vi "Instrument Manager Loop.vi"(8 "System Control":refnum<queue>, 11 "Instrument Manager":refnum<queue>) -> (0 "error out":errorcluster)   [LabVIEW 2020, in "plugin_flodx_ph_probe.lvlib" / "plugin.lvlib" / "Instrument Manager.lvlib"]
uses:
  Instrument Manager.lvlib
  <userlib>/RxnRover/PluginCore/src/support/Message Queue/Message Cluster.ctl
  Instrument Loop State.ctl
  connection_info/Connection Info.ctl
  Instrument State.ctl
  Instrument Config.ctl
  <vilib>/Utility/error.llb/Error Cluster From Error Code.vi
  <vilib>/ErrorRing/Error Ring.xnode
  <userlib>/RxnRover/PluginCore/src/support/Message Queue/Message Queue.lvlib
  <userlib>/_OpenG.lib/lvdata/lvdata.llb/openg_variant.lvlib
  mock_driver/mock_driver.lvlib
  <instrlib>/RxnRover/FloDx Ph Probe Driver/driver_flodx_ph_probe.lvlib
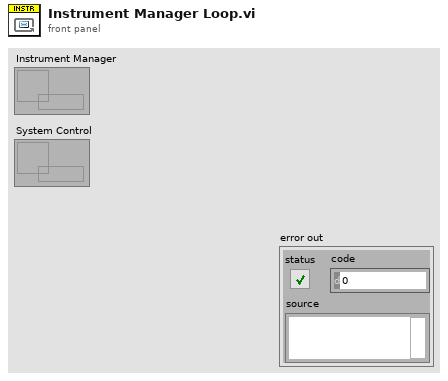
[diagram p1: front panel]
types:
  T1 = typedef "plugin_flodx_ph_probe.lvlib/plugin.lvlib/Instrument Manager.lvlib/Instrument Loop State.ctl" = cluster{"Connection Info":T2, "Running":bool, "Running Since":timestamp, "Instrument State":T3}
  T2 = typedef "plugin_flodx_ph_probe.lvlib/plugin.lvlib/Instrument Manager.lvlib/Connection Info.ctl" = cluster{"VISA Resource":refnum<visa-resource-name>, "Address":u8}
  T3 = typedef "plugin_flodx_ph_probe.lvlib/plugin.lvlib/Instrument Manager.lvlib/Instrument State.ctl" = cluster{"pH":sgl, "Temperature (C)":sgl, "Device":string, "Firmware Version":string, "Error Status":bool, "Error Code":i32, "Error Source":string}
  T4 = typedef "plugin_flodx_ph_probe.lvlib/plugin.lvlib/Instrument Manager.lvlib/Instrument Config.ctl" = cluster{"Address":dbl, "Device":string, "Firmware Version":string}
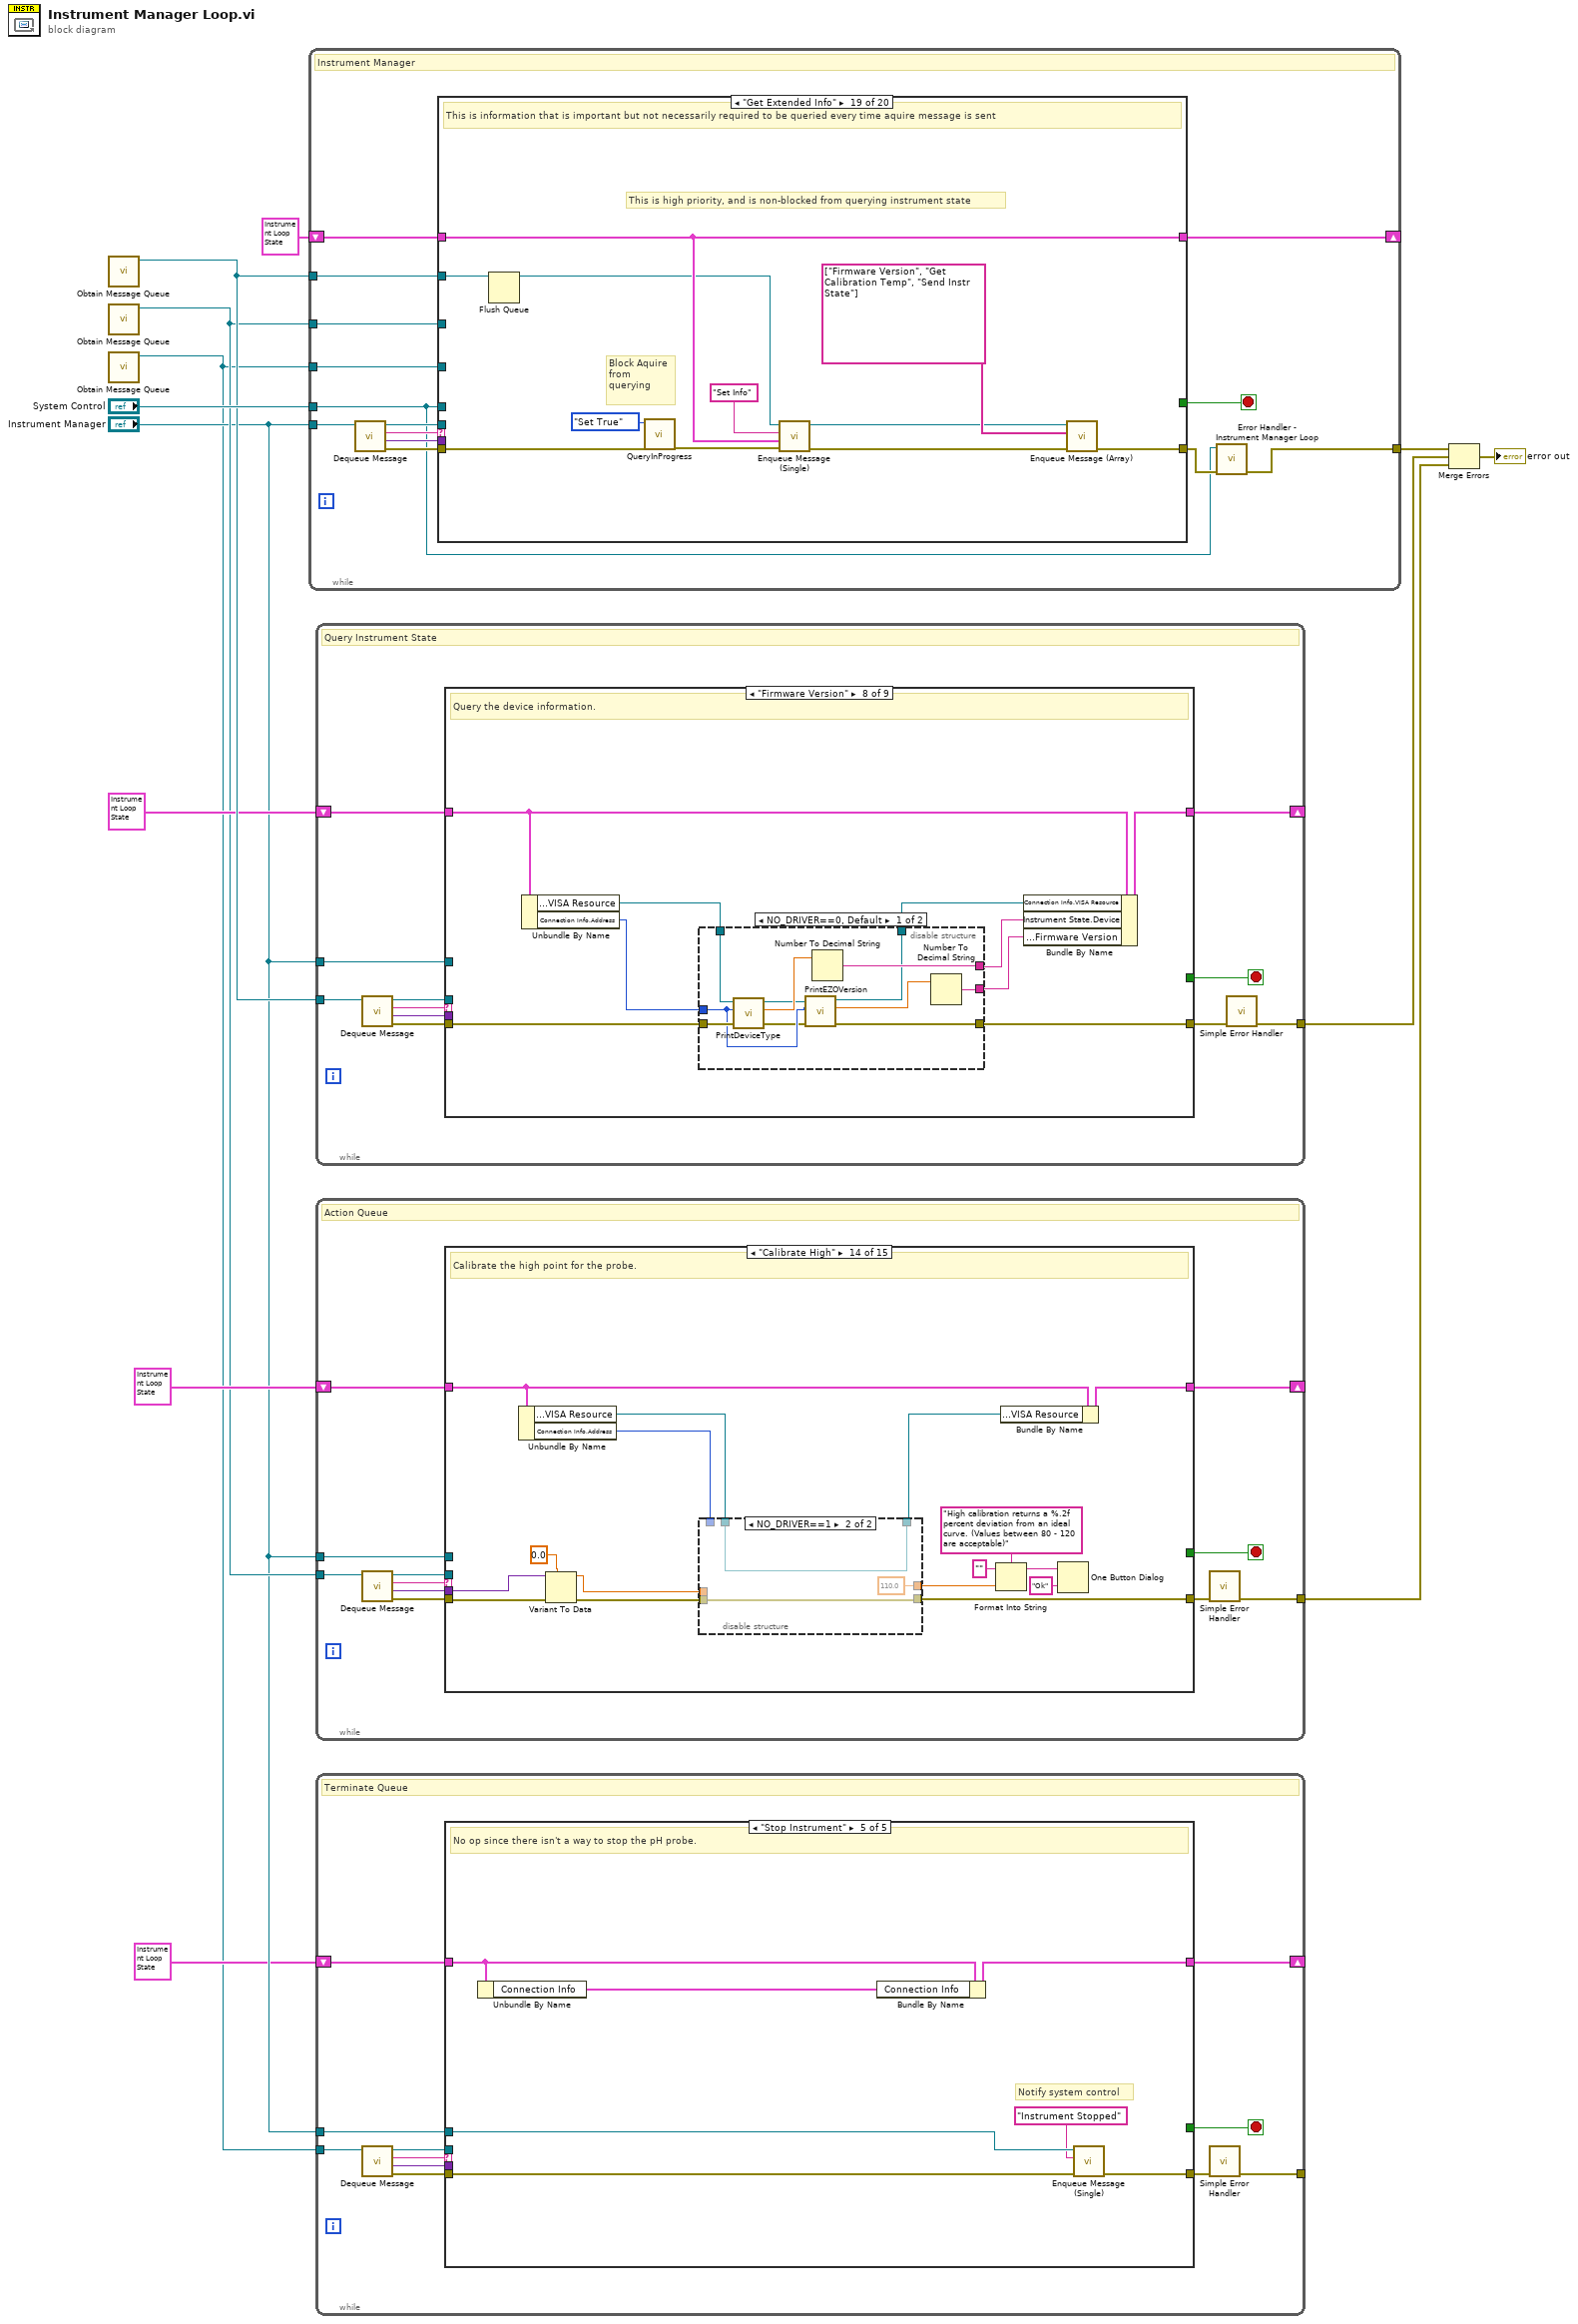
[diagram p0: block diagram]
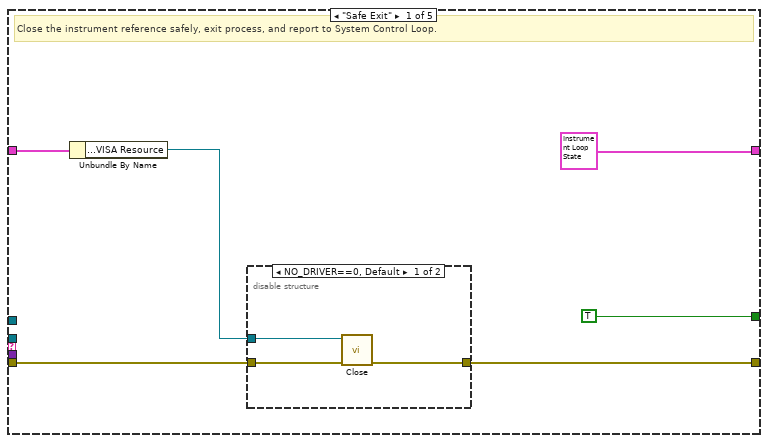
[diagram p2: hidden frame]
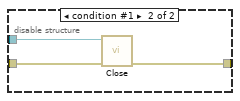
[diagram p3: hidden frame]
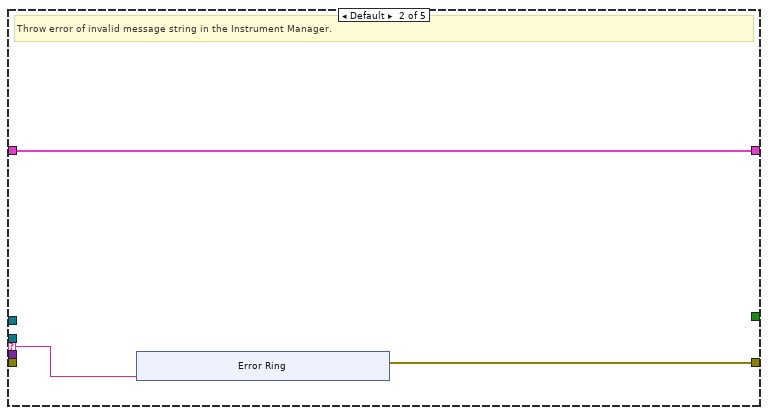
[diagram p4: hidden frame]
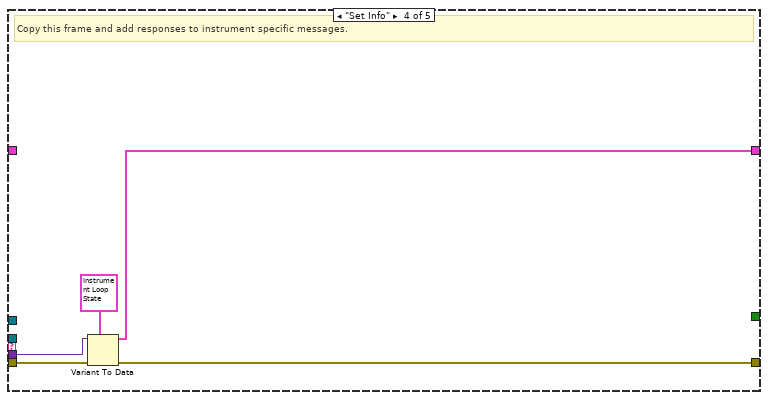
[diagram p6: hidden frame]
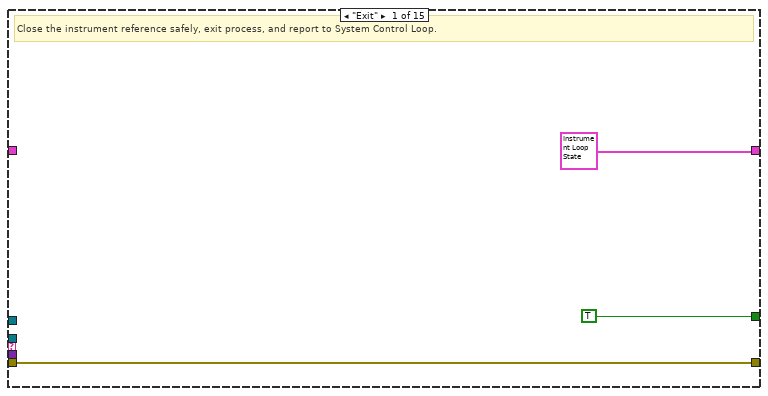
[diagram p7: hidden frame]
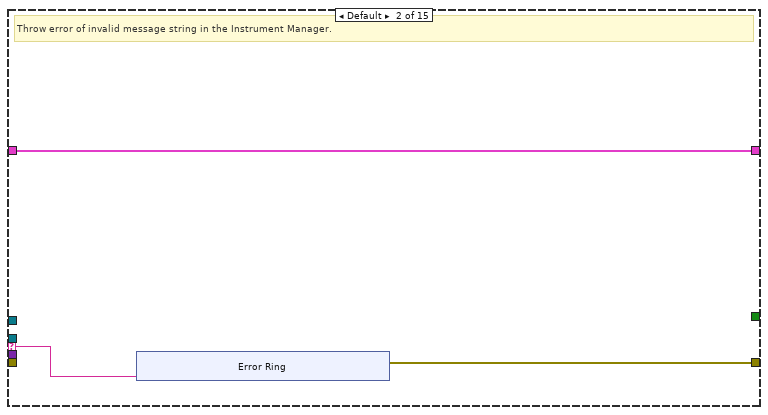
[diagram p8: hidden frame]
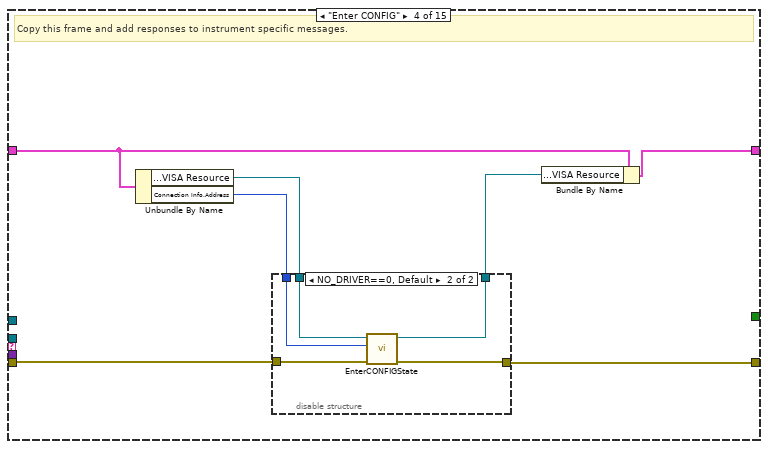
[diagram p10: hidden frame]
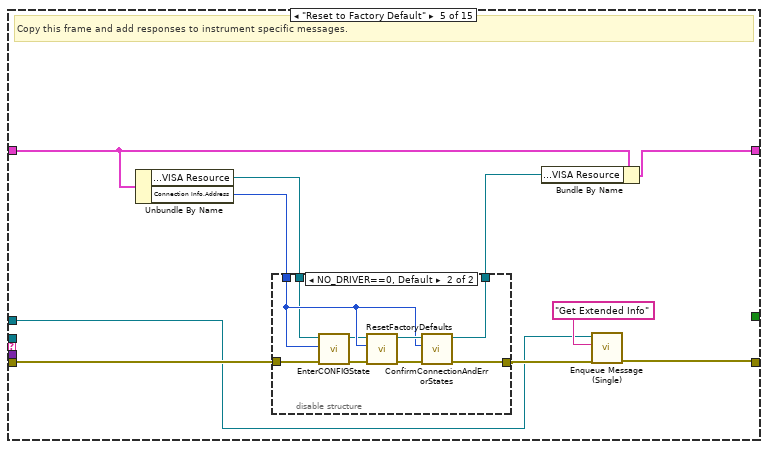
[diagram p12: hidden frame]
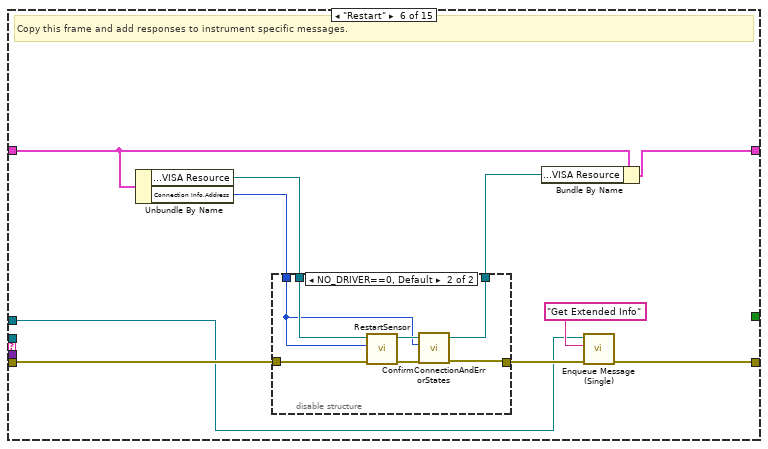
[diagram p14: hidden frame]
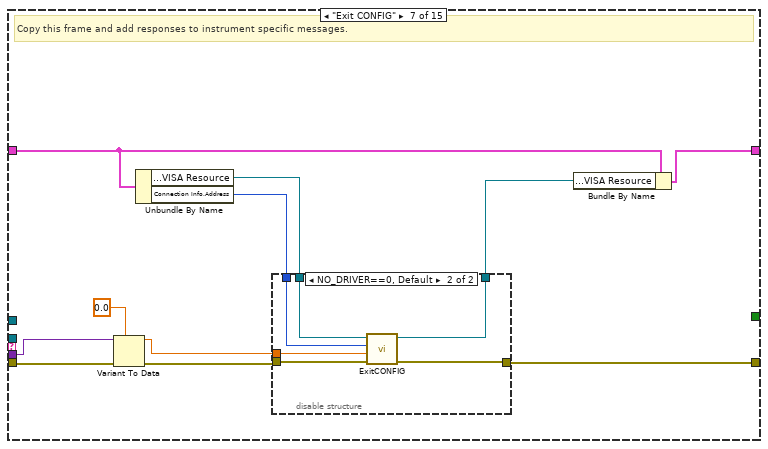
[diagram p16: hidden frame]
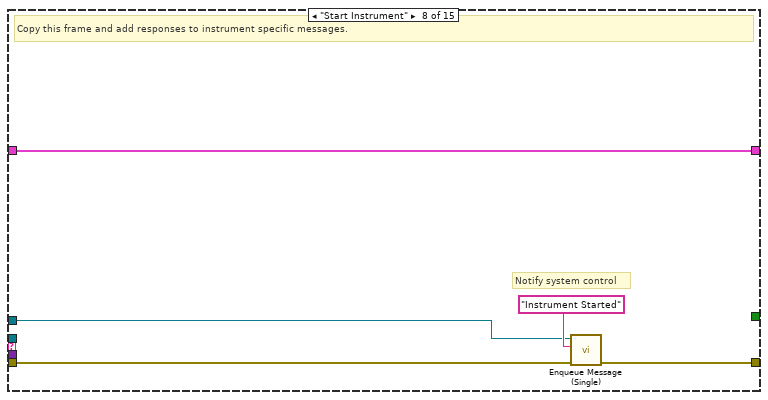
[diagram p18: hidden frame]
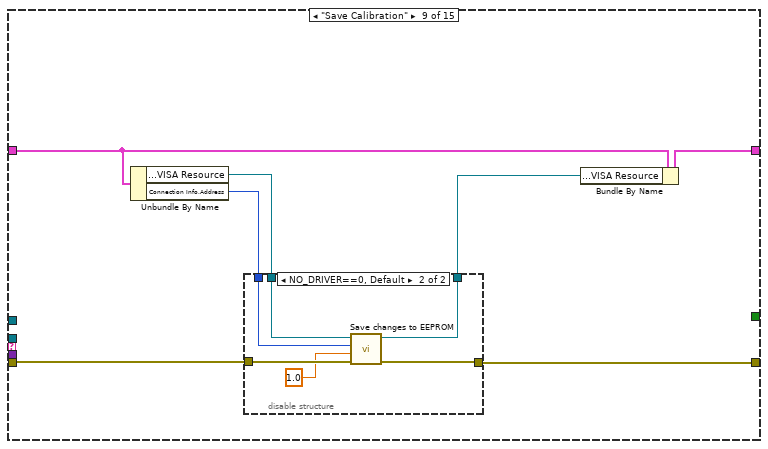
[diagram p19: hidden frame]
diagram:
  n1 = call <userlib>:"Obtain Message Queue.vi"() -> ("Message Queue"=w10:refnum<queue>)  [unwired: 10 in, 1 out]
  n2 = call <userlib>:"Obtain Message Queue.vi"() -> ("Message Queue"=w5:refnum<queue>)  [unwired: 10 in, 1 out]
  n3 = call <userlib>:"Obtain Message Queue.vi"() -> ("Message Queue"=w1:refnum<queue>)  [unwired: 10 in, 1 out]
  n4 = while {
    tunnel: "Instrument Manager" -> [w27]
    tunnel: "System Control" -> [w18]
    tunnel: [w21] -> w13
    shift-right: [w14] -> _
    shift-left: T1 {"Connection Info"={"VISA Resource"="", "Address"=0}, "Running"=FALSE, "Running Since"=timestamp(0 s since 1904-01-01), "Instrument State"={"pH"=0.0, "Temperature (C)"=0.0, "Device"="", "Firmware Version"="", "Error Status"=FALSE, "Error Code"=0, "Error Source"=""}} ("Default Instrument State") -> [w20]
    tunnel: w10 -> [w17]
    tunnel: w5 -> [w16]
    tunnel: w1 -> [w15]
    stop <- w19 stop-if-true
    # "Instrument Manager"
    n5 = call <userlib>:"Dequeue Message.vi"("Message Queue"=w27) -> ("error out"=w23:errorcluster, "Message Data"=w24:variant, "Message"=w26:string, "dup Message Queue"=w25:refnum<queue>)  [unwired: 7 in]
    n6 = case shown="\"Get Extended Info\"" w26 {
      selector: w26 -> [_ w37 _ _ _ _ _ w83 _ _ w128 w132 w145 w154 w164 w176 _ _ _ _]
      tunnel: w25 -> [w30 _ _ w54 _ _ _ _ _ w94 _ _ _ _ _ w174 _ _ _ w215]
      tunnel: w18 -> [_ w38 _ _ w64 w74 w80 _ _ w96 w124 _ _ _ _ _ _ _ _ _]
      tunnel: w24 -> [_ _ _ w61 _ _ _ _ _ w102 w127 w139 w151 w160 w170 w182 _ _ _ w216]
      tunnel: w23 -> [w31 w39 w46 w59 w66 w71 w77 _ w92 w101 w126 w136 w148 w157 w167 w179 w184 w185 w201 w221]
      tunnel: [w29 w33 w47 w56 w65 w75 w81 w82 w92 w105 w129 w140 w152 w161 w162 w172 w184 w191 w211 w212] -> w22
      tunnel: w20 -> [_ w36 _ w60 w67 w69 w78 w84 w93 w104 w125 w137 w149 w158 w168 w180 w183 w190 w208 w220]
      tunnel: [w32 w36 T1 {"Connection Info"={"VISA Resource"="", "Address"=0}, "Running"=FALSE, "Running Since"=timestamp(0 s since 1904-01-01), "Instrument State"={"pH"=0.0, "Temperature (C)"=0.0, "Device"="", "Firmware Version"="", "Error Status"=FALSE, "Error Code"=0, "Error Source"=""}} w60 w67 w69 w78 w84 w93 w103 w125 w131 w144 w158 w168 w180 w183 w190 w208 w214] -> w14
      tunnel: [_ _ TRUE _ _ _ _ _ _ _ _ _ _ _ _ _ _ _ _ _] -> w19
      tunnel: w17 -> [_ _ w41 _ _ _ _ _ _ _ _ _ _ _ _ _ _ w189 w203 _]
      tunnel: w16 -> [_ _ w42 _ _ _ _ _ _ _ _ _ w141 w153 w163 w175 _ _ _ _]
      tunnel: w15 -> [_ _ w43 _ _ _ _ _ _ _ _ w134 _ _ _ _ _ _ _ _]
      frame "Initialize" {
        (unwired) string[] ["Send Instrument Config", "Send Entry Names"]
        w32 = T1 {"Connection Info"={"VISA Resource"="", "Address"=0}, "Running"=FALSE, "Running Since"=timestamp(0 s since 1904-01-01), "Instrument State"={"pH"=0.0, "Temperature (C)"=0.0, "Device"="", "Firmware Version"="", "Error Status"=FALSE, "Error Code"=0, "Error Source"=""}}  # Default Instrument State
        # "Initialize the loop data."
        n7 = call <userlib>:"Enqueue Message (Array).vi"("error in (no error)"=w31, "Message Array"=string[] ["Send Instrument Config", "Send Acquisition Messages", "Send Entry Names"], "Message Queue"=w30) -> ("error out"=w29:errorcluster)  [unwired: 7 in, 1 out]
      }
      frame "Report" {
        # "Unblock querying"
        # "Report the instrument state."
        n8 = call <userlib>:"Enqueue Message (Single).vi"("error in (no error)"=w39, "Message Data"=w36, "Message"=w37, "Message Queue"=w38) -> ("error out"=w34:errorcluster)  [unwired: 6 in, 1 out]
        n9 = call "QueryInProgress.vi"("error in (no error)"=w34, "Action"=enum16{"Get", "Set False", "Set True"}."Set False") -> ("error out"=w33:errorcluster)  [unwired: 8 in, 1 out]
      }
      frame "Exit" {
        # "Close the instrument reference safely, exit process, and report to System Control Loop."
        n10 = Build Array(w41, w42) -> (w40:refnum<queue>[])
        n11 = call <userlib>:"Enqueue Message (Single).vi"("error in (no error)"=w46, "Message"="Safe Exit", "Message Queue"=w43) -> ("error out"=w45:errorcluster)  [unwired: 7 in, 1 out]
        n12 = for {
          tunnel: w40 -> [w52] mode=indexing
          tunnel: w45 -> [w50]
          tunnel: [w53] -> w47
          n13 = call <userlib>:"Enqueue Message (Single).vi"("error in (no error)"=w50, "Message"="Exit", "Message Queue"=w52) -> ("error out"=w53:errorcluster)  [unwired: 7 in, 1 out]
        }
      }
      frame "New Instrument Config" {
        # "No settings right now"
        # "#todo: What if values are invalid? Create \"Invalid Instrument Config\" message maybe."
        # "If the new config is accepted, notify everything of the new values"
        # "Update the configs based on the user settings."
        n14 = Variant To Data(error in=w59, type=T4 {"Address"=0.0, "Device"="", "Firmware Version"=""} ("Instrument Configuration"), Variant=w61) -> (error out=w55:errorcluster)  [unwired: 1 out]
        n15 = call <userlib>:"Enqueue Message (Single).vi"("error in (no error)"=w55, "Message"="Send Instrument Config", "Message Queue"=w54) -> ("error out"=w56:errorcluster)  [unwired: 7 in, 1 out]
      }
      frame "Send Instrument Config" {
        # "Send out the current values for the public loop configs."
        n16 = call <userlib>:"Enqueue Message (Single).vi"("error in (no error)"=w66, "Message Data"=T4 {"Address"=0.0, "Device"="", "Firmware Version"=""} ("Instrument Configuration"), "Message"="Instrument Config", "Message Queue"=w64) -> ("error out"=w65:errorcluster)  [unwired: 6 in, 1 out]
      }
      frame "Send Entry Names" {
        # "#note: This is auto-populated based on the Instrument State TypeDef entry labels."
        # "Send the display names of entry values that will be reported by this instrument in each \"Report\" call."
        n17 = Unbundle By Name(w69) -> ("Instrument State"=w68:T3)
        n18 = call <userlib>:"Get Cluster Element Names__ogtk.vi"("error in (no error)"=w71, "Cluster"=w68) -> ("error out"=w70:errorcluster, "Element Names"=w72:string[])  [unwired: 8 in]
        n19 = call <userlib>:"Enqueue Message (Single).vi"("error in (no error)"=w70, "Message Data"=w72, "Message"="Set Entry Names", "Message Queue"=w74) -> ("error out"=w75:errorcluster)  [unwired: 6 in, 1 out]
      }
      frame "Send Acquisition Messages" {
        # "Send the messages that should be used to acquire the relevant instrument state and how to report it."
        n20 = call <userlib>:"Enqueue Message (Single).vi"("error in (no error)"=w77, "Message Data"=string[] ["Acquire"], "Message"="Set Acquisition Messages", "Message Queue"=w80) -> ("error out"=w81:errorcluster)  [unwired: 6 in, 1 out]
      }
      frame Default {
        # "Throw error of invalid message string in the Instrument Manager."
        n21 = xnode "Error Ring"("parameter 0"=w83) -> ("error out"=w82:errorcluster)
      }
      frame "--- Copy This Frame ---" {
        # "Copy this frame and add responses to instrument specific messages."
      }
      frame "Set Connection Info" {
        # "Validate and initialize the connection info"
        n22 = Variant To Data(error in=w101, type=T2 {"VISA Resource"="", "Address"=0} ("Connection Info"), Variant=w102) -> (data=w99:T2, error out=w100:errorcluster)
        n23 = call "Attempt Connection.vi"("error in (no error)"=w100, "Connection Info"=w99) -> ("error out"=w97:errorcluster, "Connection Info (duplicate)"=w98:T2)  [unwired: 8 in]
        n24 = case shown="No Error" w97 {
          selector: w97 -> [w107 w119]
          tunnel: w98 -> [w106 _]
          tunnel: [w108 w122] -> w105
          tunnel: w104 -> [w115 w123]
          tunnel: [w117 w123] -> w103
          tunnel: w96 -> [w116 w121]
          tunnel: w94 -> [w112 _]
          frame No Error {
            # "Notify System Control of valid connection info"
            # "Initialize valid resource."
            n25 = call <userlib>:"Enqueue Message (Single).vi"("error in (no error)"=w107, "Message Data"=w106, "Message"="Valid Connection Info", "Message Queue"=w116) -> ("error out"=w114:errorcluster)  [unwired: 6 in, 1 out]
            n26 = Bundle By Name(cluster=w115, "Connection Info"=w106) -> (w117:T1)
            n27 = call <userlib>:"Enqueue Message (Single).vi"("error in (no error)"=w114, "Message"="Send Acquisition Messages", "Message Queue"=w112) -> ("error out"=w109:errorcluster, "dup Message Queue"=w111:refnum<queue>)  [unwired: 7 in]
            n28 = call <userlib>:"Enqueue Message (Single).vi"("error in (no error)"=w109, "Message"="Get Extended Info", "Message Queue"=w111) -> ("error out"=w108:errorcluster)  [unwired: 7 in, 1 out]
          }
          frame Error {
            # "Report invalid resource."
            n29 = call <userlib>:"Enqueue Message (Single).vi"("Message Data"=w119, "Message"="Invalid Connection Info", "Message Queue"=w121) -> ("error out"=w122:errorcluster)  [unwired: 7 in, 1 out]
          }
        }
      }
      frame "Instrument Started", "Instrument Stopped" {
        # "Forward start/stop messages to the rest of the program."
        n30 = call <userlib>:"Enqueue Message (Single).vi"("error in (no error)"=w126, "Message Data"=w127, "Message"=w128, "Message Queue"=w124) -> ("error out"=w129:errorcluster)  [unwired: 6 in, 1 out]
      }
      frame "Stop Instrument" {
        # "Stop the instrument action."
        n31 = call <userlib>:"Enqueue Message (Single).vi"("error in (no error)"=w136, "Message Data"=w137, "Message"="Set Info", "Message Queue"=w134) -> ("error out"=w135:errorcluster, "dup Message Queue"=w133:refnum<queue>)  [unwired: 6 in]
        n32 = call <userlib>:"Enqueue Message (Single).vi"("error in (no error)"=w135, "Message Data"=w139, "Message"=w132, "Message Queue"=w133) -> ("error out"=w140:errorcluster)  [unwired: 6 in, 1 out]
        n33 = Bundle By Name(cluster=w137, "Running"=FALSE) -> (w131:T1)
      }
      frame "Start Instrument" {
        # "Start the instrument action."
        n34 = call <userlib>:"Enqueue Message (Single).vi"("error in (no error)"=w148, "Message Data"=w149, "Message"="Set Info", "Message Queue"=w141) -> ("error out"=w147:errorcluster, "dup Message Queue"=w146:refnum<queue>)  [unwired: 6 in]
        n35 = call <userlib>:"Enqueue Message (Single).vi"("error in (no error)"=w147, "Message Data"=w151, "Message"=w145, "Message Queue"=w146) -> ("error out"=w152:errorcluster)  [unwired: 6 in, 1 out]
        n36 = Get Date/Time In Seconds() -> (seconds since 1Jan1904=w142:timestamp)
        n37 = Bundle By Name(cluster=w149, "Running"=TRUE, "Running Since"=w142) -> (w144:T1)
      }
      frame "Calibrate High", "Calibrate Low", "Calibrate Mid", "Clear Calibration", "Enter CONFIG", "Exit CONFIG", "Set Address", "Set Compensation Temperature" {
        # "Actions to be forwarded to the Action loop"
        n38 = call <userlib>:"Enqueue Message (Single).vi"("error in (no error)"=w157, "Message Data"=w158, "Message"="Set Info", "Message Queue"=w153) -> ("error out"=w156:errorcluster, "dup Message Queue"=w155:refnum<queue>)  [unwired: 6 in]
        n39 = call <userlib>:"Enqueue Message (Single).vi"("error in (no error)"=w156, "Message Data"=w160, "Message"=w154, "Message Queue"=w155) -> ("error out"=w161:errorcluster)  [unwired: 6 in, 1 out]
      }
      frame "Reset to Factory Default", "Restart" {
        # "On Reset and Restart  device info will need to be queried again"
        n40 = call <userlib>:"Enqueue Message (Single).vi"("error in (no error)"=w167, "Message Data"=w168, "Message"="Set Info", "Message Queue"=w163) -> ("error out"=w166:errorcluster, "dup Message Queue"=w165:refnum<queue>)  [unwired: 6 in]
        n41 = call <userlib>:"Enqueue Message (Single).vi"("error in (no error)"=w166, "Message Data"=w170, "Message"=w164, "Message Queue"=w165) -> ("error out"=w162:errorcluster)  [unwired: 6 in, 1 out]
      }
      frame "Save Calibration" {
        # "Actions to be forwarded to the Action loop"
        n42 = call <userlib>:"Enqueue Message (Single).vi"("error in (no error)"=w179, "Message Data"=w180, "Message"="Set Info", "Message Queue"=w175) -> ("error out"=w178:errorcluster, "dup Message Queue"=w177:refnum<queue>)  [unwired: 6 in]
        n43 = call <userlib>:"Enqueue Message (Single).vi"("error in (no error)"=w178, "Message Data"=w182, "Message"=w176, "Message Queue"=w177) -> ("error out"=w173:errorcluster)  [unwired: 6 in, 1 out]
        n44 = call <userlib>:"Enqueue Message (Single).vi"("error in (no error)"=w173, "Message"="Get Extended Info", "Message Queue"=w174) -> ("error out"=w172:errorcluster)  [unwired: 7 in, 1 out]
      }
      frame "--- Copy for Get State Messages ---" {
        # "#CodeNeeded - Use the Bundle by Name function to bundle the new state value into the Instrument State cluster."
        # "#CodeNeeded - Add instrument driver call to query the instrument state requested"
        # "Duplicate this case for messages cases that will query the instrument state."
      }
      frame "Acquire" {
        # "Only query if there isn't another query in progress"
        # "Query the run state of the instrument."
        n45 = call "QueryInProgress.vi"("error in (no error)"=w185, "Action"=enum16{"Get", "Set False", "Set True"}."Get") -> ("error out"=w186:errorcluster, "Value"=w187:bool)  [unwired: 8 in]
        n46 = case shown="False" w187 {
          tunnel: w186 -> [w192 w200]
          tunnel: [w192 w199] -> w191
          tunnel: w190 -> [_ w196]
          tunnel: w189 -> [_ w194]
          frame True {
            # "There is another process inside Query Instrument\nstate, wait until it is finished"
          }
          frame False {
            n47 = call <userlib>:"Enqueue Message (Single).vi"("error in (no error)"=w200, "Message Data"=w196, "Message"="Set Info", "Message Queue"=w194) -> ("error out"=w197:errorcluster, "dup Message Queue"=w193:refnum<queue>)  [unwired: 6 in]
            n48 = call <userlib>:"Enqueue Message (Array).vi"("error in (no error)"=w197, "Message Array"=string[] ["pH", "Send Instr State"], "Message Queue"=w193) -> ("error out"=w199:errorcluster)  [unwired: 7 in, 1 out]
          }
        }
      }
      frame "Get Extended Info" {
        # "Block Aquire from querying"
        # "This is high priority, and is non-blocked from querying instrument state"
        # "This is information that is important but not necessarily required to be queried every time aquire message is sent"
        n49 = Flush Queue(queue=w203) -> (queue out=w202:refnum<queue>)  [unwired: 1 in, 2 out]
        n50 = call "QueryInProgress.vi"("error in (no error)"=w201, "Action"=enum16{"Get", "Set False", "Set True"}."Set True") -> ("error out"=w204:errorcluster)  [unwired: 8 in, 1 out]
        n51 = call <userlib>:"Enqueue Message (Single).vi"("error in (no error)"=w204, "Message Data"=w208, "Message"="Set Info", "Message Queue"=w202) -> ("error out"=w209:errorcluster, "dup Message Queue"=w206:refnum<queue>)  [unwired: 6 in]
        n52 = call <userlib>:"Enqueue Message (Array).vi"("error in (no error)"=w209, "Message Array"=string[] ["Firmware Version", "Get Calibration Temp", "Send Instr State"], "Message Queue"=w206) -> ("error out"=w211:errorcluster)  [unwired: 7 in, 1 out]
      }
      frame "Set Instr State" {
        # "Set the new instrument state queried from the instrument."
        n53 = Variant To Data(error in=w221, type=T3 {"pH"=0.0, "Temperature (C)"=0.0, "Device"="", "Firmware Version"="", "Error Status"=FALSE, "Error Code"=0, "Error Source"=""} ("Instrument State"), Variant=w216) -> (data=w213:T3, error out=w218:errorcluster)
        n54 = Bundle By Name(cluster=w220, "Instrument State"=w213) -> (w214:T1)
        n55 = call <userlib>:"Enqueue Message (Single).vi"("error in (no error)"=w218, "Message"="Report", "Message Queue"=w215) -> ("error out"=w212:errorcluster)  [unwired: 7 in, 1 out]
      }
    }
    n56 = call "Error Handler - Instrument Manager Loop.vi"("error in (no error)"=w22, "Message Queue"=w18) -> ("dup error in"=w21:errorcluster)  [unwired: 8 in, 1 out]
  }
  n57 = while {
    tunnel: w10 -> [w232]
    shift-right: [w226] -> _
    shift-left: T1 {"Connection Info"={"VISA Resource"="", "Address"=0}, "Running"=FALSE, "Running Since"=timestamp(0 s since 1904-01-01), "Instrument State"={"pH"=0.0, "Temperature (C)"=0.0, "Device"="", "Firmware Version"="", "Error Status"=FALSE, "Error Code"=0, "Error Source"=""}} ("Default Instrument State") -> [w227]
    tunnel: "Instrument Manager" -> [w224]
    tunnel: [w222] -> w7
    stop <- w225 stop-if-true
    # "Query Instrument State"
    n58 = call <userlib>:"Dequeue Message.vi"("Message Queue"=w232) -> ("error out"=w228:errorcluster, "Message Data"=w229:variant, "Message"=w231:string, "dup Message Queue"=w230:refnum<queue>)  [unwired: 7 in]
    n59 = case shown="\"Firmware Version\"" w231 {
      selector: w231 -> [_ w237 _ _ _ _ _ _ _]
      tunnel: w230 -> [_ _ _ _ _ _ _ _ _]
      tunnel: w229 -> [_ _ _ _ w253 _ _ _ _]
      tunnel: w228 -> [w233 _ w247 w250 w255 w261 w280 w298 w321]
      tunnel: [w233 w236 w247 w250 w254 w260 w279 w297 w316] -> w223
      tunnel: w227 -> [_ w238 w248 w249 _ w262 w281 w299 w319]
      tunnel: [T1 {"Connection Info"={"VISA Resource"="", "Address"=0}, "Running"=FALSE, "Running Since"=timestamp(0 s since 1904-01-01), "Instrument State"={"pH"=0.0, "Temperature (C)"=0.0, "Device"="", "Firmware Version"="", "Error Status"=FALSE, "Error Code"=0, "Error Source"=""}} w238 w248 w249 w251 w263 w282 w300 w319] -> w226
      tunnel: [TRUE _ _ _ _ _ _ _ _] -> w225
      tunnel: w224 -> [_ _ _ _ _ _ _ _ w320]
      frame "Exit" {
        # "Close the instrument reference safely, exit process, and report to System Control Loop."
      }
      frame Default {
        # "Throw error of invalid message string in the Instrument Manager."
        n60 = xnode "Error Ring"("parameter 0"=w237) -> ("error out"=w236:errorcluster)
      }
      frame "Wait" {
        # "Simply waits for a designated amount of time, useful for timing/synchronization."
        n61 = Wait (ms)(milliseconds to wait=u32 2000) -> ()  [unwired: 1 out]
      }
      frame "--- Copy for Get State Messages ---" {
        # "#CodeNeeded - Use the Bundle by Name function to bundle the new state value into the Instrument State cluster."
        # "#CodeNeeded - Add instrument driver call to query the instrument state requested"
        # "Duplicate this case for messages cases that will query the instrument state."
      }
      frame "Set Info" {
        # "Sets the instrument loop info needed for operation."
        n62 = Variant To Data(error in=w255, type=T1 {"Connection Info"={"VISA Resource"="", "Address"=0}, "Running"=FALSE, "Running Since"=timestamp(0 s since 1904-01-01), "Instrument State"={"pH"=0.0, "Temperature (C)"=0.0, "Device"="", "Firmware Version"="", "Error Status"=FALSE, "Error Code"=0, "Error Source"=""}} ("Default Instrument State"), Variant=w253) -> (data=w251:T1, error out=w254:errorcluster)
      }
      frame "pH" {
        # "Query the pH reading of the probe."
        n63 = Unbundle By Name(w262) -> ("Connection Info.VISA Resource"=w259:refnum<visa-resource-name>, "Connection Info.Address"=w256:u8)
        n64 = disable-structure shown="NO_DRIVER==1" {
          disable-tunnel: w261 -> [w269 w274]
          disable-tunnel: [w265 w273] -> w260
          disable-tunnel: w259 -> [w268 w272]
          disable-tunnel: [w267 w271] -> w258
          disable-tunnel: [w266 w270] -> w257
          disable-tunnel: w256 -> [w264 _]
          frame condition #0 (active) {
            n65 = call <instrlib>:"PrintpH.vi"("error in (no error)"=w269, "Address"=w264, "VISA resource name"=w268) -> ("error out"=w265:errorcluster, "pH"=w266:dbl, "VISA resource name out"=w267:refnum<visa-resource-name>)  [unwired: 5 in, 1 out]
          }
          frame condition #1 {
            n66 = call "Status pH.vi"("error in (no error)"=w274, "VISA Resource in"=w272) -> ("error out"=w273:errorcluster, "pH"=w270:dbl, "VISA Resource out"=w271:refnum<visa-resource-name>)  [unwired: 7 in]
          }
        }
        n67 = Bundle By Name(cluster=w262, "Connection Info.VISA Resource"=w258, "Instrument State.pH"=w257) -> (w263:T1)
      }
      frame "Get Calibration Temp" {
        # "Query the compensated temperature value of the probe."
        n68 = Unbundle By Name(w281) -> ("Connection Info.VISA Resource"=w278:refnum<visa-resource-name>, "Connection Info.Address"=w275:u8)
        n69 = disable-structure shown="NO_DRIVER==1" {
          disable-tunnel: w280 -> [w288 w291]
          disable-tunnel: [w287 w291] -> w279
          disable-tunnel: w278 -> [w285 w290]
          disable-tunnel: [w284 w290] -> w277
          disable-tunnel: [w286 sgl 15.0 ("Temp")] -> w276
          disable-tunnel: w275 -> [w283 _]
          frame condition #0 (active) {
            n70 = call <instrlib>:"PrintCompensationTemperature.vi"("error in (no error)"=w288, "Address"=w283, "VISA resource name"=w285) -> ("error out"=w287:errorcluster, "Temp"=w286:dbl, "VISA resource name out"=w284:refnum<visa-resource-name>)  [unwired: 5 in, 1 out]
          }
          frame condition #1 {
          }
        }
        n71 = Bundle By Name(cluster=w281, "Connection Info.VISA Resource"=w277, "Instrument State.Temperature (C)"=w276) -> (w282:T1)
      }
      frame "Firmware Version" {
        # "Query the device information."
        n72 = Unbundle By Name(w299) -> ("Connection Info.VISA Resource"=w296:refnum<visa-resource-name>, "Connection Info.Address"=w292:u8)
        n73 = disable-structure shown="NO_DRIVER==0, Default" {
          disable-tunnel: w298 -> [w311 w315]
          disable-tunnel: [w304 w315] -> w297
          disable-tunnel: w296 -> [w310 w314]
          disable-tunnel: [w303 w314] -> w295
          disable-tunnel: [w308 "mock"] -> w294
          disable-tunnel: [w301 "123"] -> w293
          disable-tunnel: w292 -> [w306 _]
          frame condition #0 (active) {
            n74 = call <instrlib>:"PrintDeviceType.vi"("error in (no error)"=w311, "Address"=w306, "VISA resource name"=w310) -> ("error out"=w305:errorcluster, "Device Type"=w309:dbl, "VISA resource name out"=w307:refnum<visa-resource-name>)  [unwired: 5 in, 1 out]
            n75 = call <instrlib>:"PrintEZOVersion.vi"("error in"=w305, "Address"=w306, "VISA resource name"=w307) -> ("error out"=w304:errorcluster, "EZO Version"=w302:dbl, "VISA resource name out"=w303:refnum<visa-resource-name>)  [unwired: 5 in, 1 out]
            n76 = Number To Decimal String(number=w309) -> (decimal integer string=w308:string)  [unwired: 1 in]
            n77 = Number To Decimal String(number=w302) -> (decimal integer string=w301:string)  [unwired: 1 in]
          }
          frame condition #1 {
          }
        }
        n78 = Bundle By Name(cluster=w299, "Connection Info.VISA Resource"=w295, "Instrument State.Device"=w294, "Instrument State.Firmware Version"=w293) -> (w300:T1)
      }
      frame "Send Instr State" {
        # "Send the instrument state back to the control loop."
        n79 = Unbundle By Name(w319) -> ("Instrument State"=w318:T3)
        n80 = call <userlib>:"Enqueue Message (Single).vi"("error in (no error)"=w321, "Message Data"=w318, "Message"="Set Instr State", "Message Queue"=w320) -> ("error out"=w316:errorcluster)  [unwired: 6 in, 1 out]
      }
    }
    n81 = call <vilib>:"Simple Error Handler.vi"("error in (no error)"=w223) -> ("error out"=w222:errorcluster)  [unwired: 4 in, 4 out]
  }
  n82 = while {
    tunnel: w5 -> [w332]
    tunnel: "Instrument Manager" -> [w323]
    tunnel: [w322] -> w4
    shift-right: [w325] -> _
    shift-left: T1 {"Connection Info"={"VISA Resource"="", "Address"=0}, "Running"=FALSE, "Running Since"=timestamp(0 s since 1904-01-01), "Instrument State"={"pH"=0.0, "Temperature (C)"=0.0, "Device"="", "Firmware Version"="", "Error Status"=FALSE, "Error Code"=0, "Error Source"=""}} ("Default Instrument State") -> [w326]
    stop <- w324 stop-if-true
    # "Action Queue"
    n83 = call <userlib>:"Dequeue Message.vi"("Message Queue"=w332) -> ("error out"=w328:errorcluster, "Message Data"=w329:variant, "Message"=w331:string, "dup Message Queue"=w330:refnum<queue>)  [unwired: 7 in]
    n84 = case shown="\"Calibrate High\"" w331 {
      selector: w331 -> [_ w337 _ _ _ _ _ _ _ _ _ _ _ _ _]
      tunnel: w330 -> [_ _ _ _ _ _ _ _ _ _ _ _ _ _ _]
      tunnel: w323 -> [_ _ _ _ w362 w383 _ w420 _ _ _ _ _ _ _]
      tunnel: w329 -> [_ _ _ _ _ _ w406 _ _ w443 w460 w473 w498 w524 _]
      tunnel: w328 -> [w333 _ w346 w353 w371 w392 w407 w421 w431 w444 w462 w472 w499 w525 w546]
      tunnel: [w333 w336 w346 w354 w363 w385 w411 w422 w430 w448 w461 w474 w500 w526 w545] -> w327
      tunnel: w326 -> [_ w338 w347 w350 w368 w389 w402 w424 w429 w450 _ w479 w505 w531 w548]
      tunnel: [T1 {"Connection Info"={"VISA Resource"="", "Address"=0}, "Running"=FALSE, "Running Since"=timestamp(0 s since 1904-01-01), "Instrument State"={"pH"=0.0, "Temperature (C)"=0.0, "Device"="", "Firmware Version"="", "Error Status"=FALSE, "Error Code"=0, "Error Source"=""}} w338 w347 w349 w367 w388 w403 w424 w428 w449 w459 w478 w504 w530 w547] -> w325
      tunnel: [TRUE _ _ _ _ _ _ _ _ _ _ _ _ _ _] -> w324
      frame "Exit" {
        # "Close the instrument reference safely, exit process, and report to System Control Loop."
      }
      frame Default {
        # "Throw error of invalid message string in the Instrument Manager."
        n85 = xnode "Error Ring"("parameter 0"=w337) -> ("error out"=w336:errorcluster)
      }
      frame "--- Copy This Frame ---" {
        # "Copy this frame and add responses to instrument specific messages."
      }
      frame "Enter CONFIG" {
        # "Copy this frame and add responses to instrument specific messages."
        n86 = Unbundle By Name(w350) -> ("Connection Info.VISA Resource"=w352:refnum<visa-resource-name>, "Connection Info.Address"=w351:u8)
        n87 = disable-structure shown="NO_DRIVER==0, Default" {
          disable-tunnel: w353 -> [w355 w361]
          disable-tunnel: [w355 w360] -> w354
          disable-tunnel: [w356 w359] -> w348
          disable-tunnel: w352 -> [w356 w358]
          disable-tunnel: w351 -> [_ w357]
          frame condition #0 {
          }
          frame condition #1 (active) {
            n88 = call <instrlib>:"EnterCONFIGState.vi"("error in (no error)"=w361, "Address"=w357, "VISA resource name"=w358) -> ("error out"=w360:errorcluster, "VISA resource name out"=w359:refnum<visa-resource-name>)  [unwired: 5 in, 2 out]
          }
        }
        n89 = Bundle By Name(cluster=w350, "Connection Info.VISA Resource"=w348) -> (w349:T1)
      }
      frame "Reset to Factory Default" {
        # "Copy this frame and add responses to instrument specific messages."
        n90 = Unbundle By Name(w368) -> ("Connection Info.VISA Resource"=w370:refnum<visa-resource-name>, "Connection Info.Address"=w369:u8)
        n91 = disable-structure shown="NO_DRIVER==0, Default" {
          disable-tunnel: w371 -> [w372 w377]
          disable-tunnel: [w372 w380] -> w364
          disable-tunnel: [w373 w379] -> w366
          disable-tunnel: w370 -> [w373 w374]
          disable-tunnel: w369 -> [_ w376]
          frame condition #0 {
          }
          frame condition #1 (active) {
            n92 = call <instrlib>:"EnterCONFIGState.vi"("error in (no error)"=w377, "Address"=w376, "VISA resource name"=w374) -> ("error out"=w378:errorcluster, "VISA resource name out"=w375:refnum<visa-resource-name>)  [unwired: 5 in, 2 out]
            n93 = call <instrlib>:"ResetFactoryDefaults.vi"("error in (no error)"=w378, "Address"=w376, "VISA resource name"=w375) -> ("error out"=w382:errorcluster, "VISA resource name out"=w381:refnum<visa-resource-name>)  [unwired: 7 in]
            n94 = call <instrlib>:"ConfirmConnectionAndErrorStates.vi"("error in (no error)"=w382, "Address"=w376, "VISA resource name"=w381) -> ("error out"=w380:errorcluster, "VISA resource name out"=w379:refnum<visa-resource-name>)  [unwired: 5 in, 2 out]
          }
        }
        n95 = Bundle By Name(cluster=w368, "Connection Info.VISA Resource"=w366) -> (w367:T1)
        n96 = call <userlib>:"Enqueue Message (Single).vi"("error in (no error)"=w364, "Message"="Get Extended Info", "Message Queue"=w362) -> ("error out"=w363:errorcluster)  [unwired: 7 in, 1 out]
      }
      frame "Restart" {
        # "Copy this frame and add responses to instrument specific messages."
        n97 = Unbundle By Name(w389) -> ("Connection Info.VISA Resource"=w391:refnum<visa-resource-name>, "Connection Info.Address"=w390:u8)
        n98 = disable-structure shown="NO_DRIVER==0, Default" {
          disable-tunnel: w392 -> [w393 w400]
          disable-tunnel: [w393 w396] -> w384
          disable-tunnel: [w394 w397] -> w387
          disable-tunnel: w391 -> [w394 w399]
          disable-tunnel: w390 -> [_ w395]
          frame condition #0 {
          }
          frame condition #1 (active) {
            n99 = call <instrlib>:"RestartSensor.vi"("error in (no error)"=w400, "Address"=w395, "VISA resource name"=w399) -> ("error out"=w398:errorcluster, "VISA resource name out"=w397:refnum<visa-resource-name>)  [unwired: 7 in]
            n100 = call <instrlib>:"ConfirmConnectionAndErrorStates.vi"("error in (no error)"=w398, "Address"=w395, "VISA resource name"=w397) -> ("error out"=w396:errorcluster)  [unwired: 5 in, 3 out]
          }
        }
        n101 = Bundle By Name(cluster=w389, "Connection Info.VISA Resource"=w387) -> (w388:T1)
        n102 = call <userlib>:"Enqueue Message (Single).vi"("error in (no error)"=w384, "Message"="Get Extended Info", "Message Queue"=w383) -> ("error out"=w385:errorcluster)  [unwired: 7 in, 1 out]
      }
      frame "Exit CONFIG" {
        # "Copy this frame and add responses to instrument specific messages."
        n103 = Variant To Data(error in=w407, type=sgl 0.0, Variant=w406) -> (data=w404:sgl, error out=w408:errorcluster)
        n104 = Unbundle By Name(w402) -> ("Connection Info.VISA Resource"=w410:refnum<visa-resource-name>, "Connection Info.Address"=w409:u8)
        n105 = disable-structure shown="NO_DRIVER==0, Default" {
          disable-tunnel: w408 -> [w412 w419]
          disable-tunnel: [w412 w418] -> w411
          disable-tunnel: [w413 w417] -> w401
          disable-tunnel: w410 -> [w413 w416]
          disable-tunnel: w409 -> [_ w415]
          disable-tunnel: w404 -> [_ w414]
          frame condition #0 {
          }
          frame condition #1 (active) {
            n106 = call <instrlib>:"ExitCONFIG.vi"("error in (no error)"=w419, "(1)Save (0)Reverts"=w414, "Address"=w415, "VISA resource name"=w416) -> ("error out"=w418:errorcluster, "VISA resource name out"=w417:refnum<visa-resource-name>)  [unwired: 4 in, 2 out]
          }
        }
        n107 = Bundle By Name(cluster=w402, "Connection Info.VISA Resource"=w401) -> (w403:T1)
      }
      frame "Start Instrument" {
        # "Notify system control"
        # "Copy this frame and add responses to instrument specific messages."
        n108 = call <userlib>:"Enqueue Message (Single).vi"("error in (no error)"=w421, "Message"="Instrument Started", "Message Queue"=w420) -> ("error out"=w422:errorcluster)  [unwired: 7 in, 1 out]
      }
      frame "Save Calibration" {
        n109 = Unbundle By Name(w429) -> ("Connection Info.VISA Resource"=w426:refnum<visa-resource-name>, "Connection Info.Address"=w425:u8)
        n110 = disable-structure shown="NO_DRIVER==0, Default" {
          disable-tunnel: w431 -> [w432 w439]
          disable-tunnel: [w432 w438] -> w430
          disable-tunnel: [w433 w437] -> w427
          disable-tunnel: w426 -> [w433 w436]
          disable-tunnel: w425 -> [_ w435]
          frame condition #0 {
          }
          frame condition #1 (active) {
            n111 = call <instrlib>:"Save changes to EEPROM.vi"("error in (no error)"=w439, "(1)Save (0)Reverts"=sgl 1.0, "Address"=w435, "VISA resource name"=w436) -> ("error out"=w438:errorcluster, "VISA resource name out"=w437:refnum<visa-resource-name>)  [unwired: 4 in, 2 out]
          }
        }
        n112 = Bundle By Name(cluster=w429, "Connection Info.VISA Resource"=w427) -> (w428:T1)
      }
      frame "Set Compensation Temperature" {
        # "Copy this frame and add responses to instrument specific messages."
        n113 = Unbundle By Name(w450) -> ("Connection Info.VISA Resource"=w447:refnum<visa-resource-name>, "Connection Info.Address"=w446:u8)
        n114 = Variant To Data(error in=w444, type=sgl 0.0, Variant=w443) -> (data=w441:sgl, error out=w445:errorcluster)
        n115 = disable-structure shown="NO_DRIVER==0, Default" {
          disable-tunnel: [w456 w458] -> w448
          disable-tunnel: w447 -> [w455 w457]
          disable-tunnel: w446 -> [w454 _]
          disable-tunnel: w445 -> [w453 w458]
          disable-tunnel: w441 -> [w452 _]
          disable-tunnel: [w451 w457] -> w440
          frame condition #0 (active) {
            n116 = call <instrlib>:"SetCompensationTemperature.vi"("error in"=w453, "Temperature"=w452, "Address"=w454, "VISA resource name"=w455) -> ("error out"=w456:errorcluster, "VISA resource name out"=w451:refnum<visa-resource-name>)  [unwired: 4 in, 2 out]
          }
          frame condition #1 {
          }
        }
        n117 = Bundle By Name(cluster=w450, "Connection Info.VISA Resource"=w440) -> (w449:T1)
      }
      frame "Set Info" {
        # "Set the current pump info."
        n118 = Variant To Data(error in=w462, type=T1 {"Connection Info"={"VISA Resource"="", "Address"=0}, "Running"=FALSE, "Running Since"=timestamp(0 s since 1904-01-01), "Instrument State"={"pH"=0.0, "Temperature (C)"=0.0, "Device"="", "Firmware Version"="", "Error Status"=FALSE, "Error Code"=0, "Error Source"=""}} ("Default Instrument State"), Variant=w460) -> (data=w459:T1, error out=w461:errorcluster)
      }
      frame "Calibrate Low" {
        # "Calibrate the low point for the probe."
        n119 = Unbundle By Name(w479) -> ("Connection Info.VISA Resource"=w477:refnum<visa-resource-name>, "Connection Info.Address"=w475:u8)
        n120 = Variant To Data(error in=w472, type=sgl 0.0, Variant=w473) -> (data=w470:sgl, error out=w469:errorcluster)
        n121 = disable-structure shown="NO_DRIVER==1" {
          disable-tunnel: w477 -> [w486 w489]
          disable-tunnel: [w485 w489] -> w476
          disable-tunnel: w475 -> [w484 _]
          disable-tunnel: [w483 w488] -> w474
          disable-tunnel: w470 -> [w482 _]
          disable-tunnel: w469 -> [w481 w488]
          disable-tunnel: [w480 89.0 ("Deviation")] -> w464
          frame condition #0 (active) {
            n122 = call <instrlib>:"SetLowCalibrationPH.vi"("error in"=w481, "Calibration pH"=w482, "Address"=w484, "VISA resource name"=w486) -> ("error out"=w483:errorcluster, "Deviation"=w480:dbl, "VISA resource name out"=w485:refnum<visa-resource-name>)  [unwired: 4 in, 1 out]
          }
          frame condition #1 {
          }
        }
        n123 = Bundle By Name(cluster=w479, "Connection Info.VISA Resource"=w476) -> (w478:T1)
        n124 = Format Into String(format string="Low calibration returns a %.2f percent deviation from an ideal curve. (Values between 80 - 120 are acceptable)", initial string="", w464) -> (resulting string=w468:string)  [unwired: 1 in, 1 out]
        n125 = One Button Dialog(message=w468, button name ("OK")="Ok") -> ()  [unwired: 1 out]
      }
      frame "Calibrate Mid" {
        # "Calibrate the middle point for the probe."
        n126 = Unbundle By Name(w505) -> ("Connection Info.VISA Resource"=w496:refnum<visa-resource-name>, "Connection Info.Address"=w497:u8)
        n127 = Variant To Data(error in=w499, type=sgl 0.0, Variant=w498) -> (data=w502:sgl, error out=w501:errorcluster)
        n128 = disable-structure shown="NO_DRIVER==1" {
          disable-tunnel: w502 -> [w512 _]
          disable-tunnel: w501 -> [w511 w514]
          disable-tunnel: [w510 w514] -> w500
          disable-tunnel: w497 -> [w509 _]
          disable-tunnel: w496 -> [w508 w515]
          disable-tunnel: [w507 w515] -> w495
          disable-tunnel: [w506 5.5 ("mV measured")] -> w491
          frame condition #0 (active) {
            n129 = call <instrlib>:"SetMidCalibrationPH.vi"("error in"=w511, "Calibration pH"=w512, "Address"=w509, "VISA resource name"=w508) -> ("error out"=w510:errorcluster, "mV measured"=w506:dbl, "VISA resource name out"=w507:refnum<visa-resource-name>)  [unwired: 4 in, 1 out]
          }
          frame condition #1 {
          }
        }
        n130 = Format Into String(format string="Mid calibration returns %.2fmv", initial string="", w491) -> (resulting string=w494:string)  [unwired: 1 in, 1 out]
        n131 = Bundle By Name(cluster=w505, "Connection Info.VISA Resource"=w495) -> (w504:T1)
        n132 = One Button Dialog(message=w494, button name ("OK")="Ok") -> ()  [unwired: 1 out]
      }
      frame "Calibrate High" {
        # "Calibrate the high point for the probe."
        n133 = Unbundle By Name(w531) -> ("Connection Info.VISA Resource"=w522:refnum<visa-resource-name>, "Connection Info.Address"=w521:u8)
        n134 = Variant To Data(error in=w525, type=sgl 0.0, Variant=w524) -> (data=w528:sgl, error out=w527:errorcluster)
        n135 = disable-structure shown="NO_DRIVER==1" {
          disable-tunnel: w528 -> [w538 _]
          disable-tunnel: w527 -> [w537 w541]
          disable-tunnel: [w536 w541] -> w526
          disable-tunnel: [w535 w540] -> w523
          disable-tunnel: w522 -> [w534 w540]
          disable-tunnel: w521 -> [w533 _]
          disable-tunnel: [w532 110.0 ("Deviation")] -> w516
          frame condition #0 (active) {
            n136 = call <instrlib>:"SetHighCalibrationPH.vi"("error in"=w537, "Calibration pH"=w538, "Address"=w533, "VISA resource name"=w534) -> ("error out"=w536:errorcluster, "Deviation"=w532:dbl, "VISA resource name out"=w535:refnum<visa-resource-name>)  [unwired: 4 in, 1 out]
          }
          frame condition #1 {
          }
        }
        n137 = Format Into String(format string="High calibration returns a %.2f percent deviation from an ideal curve. (Values between 80 - 120 are acceptable)", initial string="", w516) -> (resulting string=w520:string)  [unwired: 1 in, 1 out]
        n138 = Bundle By Name(cluster=w531, "Connection Info.VISA Resource"=w523) -> (w530:T1)
        n139 = One Button Dialog(message=w520, button name ("OK")="Ok") -> ()  [unwired: 1 out]
      }
      frame "Clear Calibration" {
        # "Clear the calibration data on the probe."
        n140 = Unbundle By Name(w548) -> ("Connection Info.VISA Resource"=w543:refnum<visa-resource-name>, "Connection Info.Address"=w542:u8)
        n141 = disable-structure shown="NO_DRIVER==0, Default" {
          disable-tunnel: w546 -> [w549 w555]
          disable-tunnel: [w549 w554] -> w545
          disable-tunnel: [w550 w553] -> w544
          disable-tunnel: w543 -> [w550 w552]
          disable-tunnel: w542 -> [_ w551]
          frame condition #0 {
          }
          frame condition #1 (active) {
            n142 = call <instrlib>:"ClearCalibration.vi"("error in (no error)"=w555, "Address"=w551, "VISA resource name"=w552) -> ("error out"=w554:errorcluster, "VISA resource name out"=w553:refnum<visa-resource-name>)  [unwired: 5 in, 2 out]
          }
        }
        n143 = Bundle By Name(cluster=w548, "Connection Info.VISA Resource"=w544) -> (w547:T1)
      }
    }
    n144 = call <vilib>:"Simple Error Handler.vi"("error in (no error)"=w327) -> ("error out"=w322:errorcluster)  [unwired: 4 in, 4 out]
  }
  n145 = while {
    tunnel: "Instrument Manager" -> [w558]
    tunnel: [w557] -> _
    shift-right: [w560] -> _
    shift-left: T1 {"Connection Info"={"VISA Resource"="", "Address"=0}, "Running"=FALSE, "Running Since"=timestamp(0 s since 1904-01-01), "Instrument State"={"pH"=0.0, "Temperature (C)"=0.0, "Device"="", "Firmware Version"="", "Error Status"=FALSE, "Error Code"=0, "Error Source"=""}} ("Default Instrument State") -> [w561]
    tunnel: w1 -> [w556]
    stop <- w559 stop-if-true
    # "Terminate Queue"
    n146 = call <userlib>:"Dequeue Message.vi"("Message Queue"=w556) -> ("error out"=w563:errorcluster, "Message Data"=w564:variant, "Message"=w566:string, "dup Message Queue"=w565:refnum<queue>)  [unwired: 7 in]
    n147 = case shown="\"Stop Instrument\"" w566 {
      selector: w566 -> [_ w580 _ _ _]
      tunnel: w565 -> [_ _ _ _ _]
      tunnel: w558 -> [_ _ _ _ w601]
      tunnel: w564 -> [_ _ _ w592 _]
      tunnel: w563 -> [w569 _ w589 w594 w599]
      tunnel: [w568 w579 w589 w593 w602] -> w562
      tunnel: w561 -> [w572 w581 w590 _ w598]
      tunnel: [T1 {"Connection Info"={"VISA Resource"="", "Address"=0}, "Running"=FALSE, "Running Since"=timestamp(0 s since 1904-01-01), "Instrument State"={"pH"=0.0, "Temperature (C)"=0.0, "Device"="", "Firmware Version"="", "Error Status"=FALSE, "Error Code"=0, "Error Source"=""}} w581 w590 w591 w600] -> w560
      tunnel: [TRUE _ _ _ _] -> w559
      frame "Safe Exit" {
        # "Close the instrument reference safely, exit process, and report to System Control Loop."
        n148 = Unbundle By Name(w572) -> ("Connection Info.VISA Resource"=w567:refnum<visa-resource-name>)
        n149 = disable-structure shown="NO_DRIVER==0, Default" {
          disable-tunnel: w569 -> [w575 w578]
          disable-tunnel: [w574 w577] -> w568
          disable-tunnel: w567 -> [w573 w576]
          frame condition #0 (active) {
            n150 = call <instrlib>:"Close.vi"("error in (no error)"=w575, "VISA resource name"=w573) -> ("error out"=w574:errorcluster)  [unwired: 9 in]
          }
          frame condition #1 {
            n151 = call <instrlib>:"Close.vi"("Error in"=w578, "VISA resource name"=w576) -> ("Error out"=w577:errorcluster)  [unwired: 9 in]
          }
        }
      }
      frame Default {
        # "Throw error of invalid message string in the Instrument Manager."
        n152 = xnode "Error Ring"("parameter 0"=w580) -> ("error out"=w579:errorcluster)
      }
      frame "--- Copy This Frame ---" {
        # "Copy this frame and add responses to instrument specific messages."
      }
      frame "Set Info" {
        # "Copy this frame and add responses to instrument specific messages."
        n153 = Variant To Data(error in=w594, type=T1 {"Connection Info"={"VISA Resource"="", "Address"=0}, "Running"=FALSE, "Running Since"=timestamp(0 s since 1904-01-01), "Instrument State"={"pH"=0.0, "Temperature (C)"=0.0, "Device"="", "Firmware Version"="", "Error Status"=FALSE, "Error Code"=0, "Error Source"=""}} ("Default Instrument State"), Variant=w592) -> (data=w591:T1, error out=w593:errorcluster)
      }
      frame "Stop Instrument" {
        # "Notify system control"
        # "No op since there isn't a way to stop the pH probe."
        n154 = Unbundle By Name(w598) -> ("Connection Info"=w597:T2)
        n155 = Bundle By Name(cluster=w598, "Connection Info"=w597) -> (w600:T1)
        n156 = call <userlib>:"Enqueue Message (Single).vi"("error in (no error)"=w599, "Message"="Instrument Stopped", "Message Queue"=w601) -> ("error out"=w602:errorcluster)  [unwired: 7 in, 1 out]
      }
    }
    n157 = call <vilib>:"Simple Error Handler.vi"("error in (no error)"=w562) -> ("error out"=w557:errorcluster)  [unwired: 4 in, 4 out]
  }
  n158 = Merge Errors(w13, w7, w4) -> (→"error out":errorcluster)
